vi "Init.vi"(8 "error in (no error)":errorcluster, 11 "uService Template in":refnum<class "DAQ Sender.lvclass">) -> (0 "error out":errorcluster, 3 "uService Template out":refnum<class "DAQ Sender.lvclass">)   [LabVIEW 2020, in "TALOS.lvlib" / "DAQ Sender.lvlib" / "DAQ Sender.lvclass"]
uses:
  DAQ Sender.lvclass
  C:/LabVIEW Code/TALOS/talos/Ancestor/Ancestor/Ancestor.lvclass
  C:/LabVIEW Code/TALOS/talos/Father of all uServices/Father of all uServices/Father of all uServices.lvclass
  Interfaces/DAQ Communication/DAQ Communication.lvclass
  Ancestor/Ancestor/Ancestor.lvclass/Ancestor.ctl
  Father of all uServices/Father of all uServices/Father of all uServices.lvclass/Father of all uServices.ctl
  DAQ Sender.lvclass/DAQ Sender.ctl
  Support VIs/Generate Error.vi
  FGV/Error Memory/Get Error Description.vi
  Support VIs/Get PC name.vi
  Support VIs/Get Class Name.vi
  <vilib>/Utility/error.llb/Clear Errors.vi
  FGV/Error Memory/Error Memory Core.vi
  <vilib>/AdvancedString/Delimited String to 1D String Array.vi
  Support VIs/Circus Root Path.vi
  FGV/Error Memory/Error Crt Lvl checker.vi
  FGV/Error Memory/Error Memory Core.vi/40c8088d-b597-4017-91af-faa98e00292e.vi
  FGV/Error Memory/Error Memory Core.vi/d4a3ab98-063c-4e44-b43d-fbdcfe6c2be2.vi
  Support VIs/Global Memory.vi
  <vilib>/Utility/LVClass/Get LV Class Name.vi
  Support VIs/Is in Packed Library.vi
  Support VIs/TALOS Root path.vi
  Support VIs/Read CSV worksheet.vi
  Support VIs/Global Constants.vi
  <vilib>/Utility/error.llb/General Error Handler.vi
  Support VIs/Error Log.vi
  <vilib>/Utility/config.llb/Open Config Data.vi
  <vilib>/Utility/config.llb/Get Section Names.vi
  <vilib>/Utility/config.llb/Get Key Names.vi
  <vilib>/Utility/config.llb/Read Key.vi
  <vilib>/Utility/config.llb/Read Key (String).vi
  <vilib>/Utility/config.llb/Close Config Data.vi
  <vilib>/Utility/error.llb/Search and Replace Pattern.vi
  Father of all uServices/Father of all uServices/Father of all uServices.lvclass
  Ancestor/Ancestor/Ancestor.lvclass
  <vilib>/Comparison/Equal/Equal Functor/Equal Functor.lvclass
  TALOS.lvlib
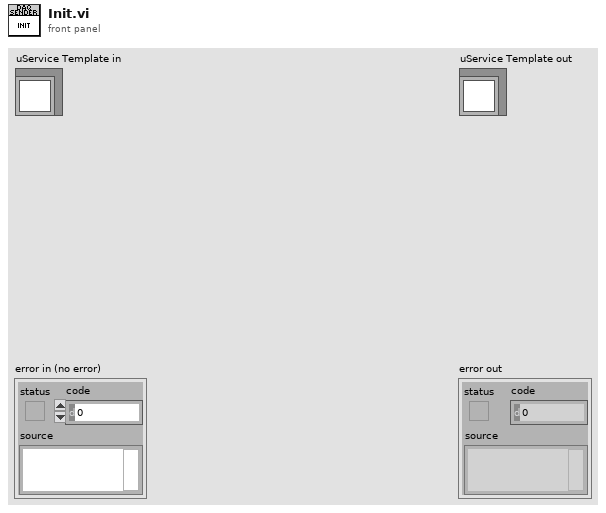
[diagram p1: front panel]
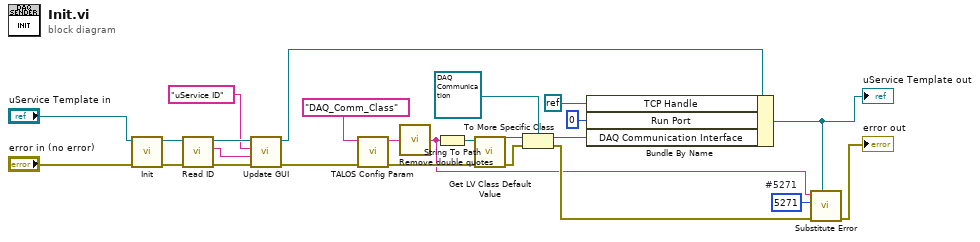
[diagram p0: block diagram]
diagram:
  w12 = 5271  # #5271
  n1 = call-parent "Init.vi"("error in (no error)"="error in (no error)", "uService Template in"="uService Template in") -> ("error out"=w21:errorcluster, "uService Template out"=w22:refnum<class "DAQ Sender.lvclass">)  [unwired: 8 in]
  n2 = call "Read ID.vi"("error in (no error)"=w21, "Ancestor in"=w22) -> ("error out"=w20:errorcluster, "ID"=w17:string, "Ancestor out"=w19:refnum<class "DAQ Sender.lvclass">)  [unwired: 7 in]
  n3 = call "Update GUI.vi"("error in (no error)"=w20, "Data"=w17, "GUI Item Name"="uService ID", "uService Template in"=w19) -> ("error out"=w1:errorcluster, "uService Template out"=w9:refnum<class "DAQ Sender.lvclass">)  [unwired: 6 in]
  n4 = call "TALOS Config Param.vi"("error in (no error)"=w1, "Parameter Name"="DAQ_Comm_Class") -> ("error out"=w25:errorcluster, "Output"=w2:string)  [unwired: 8 in]
  n5 = call "Remove double quotes.vi"("Input string"=w2) -> ("Output string"=w10:string)  [unwired: 4 in]
  n6 = String To Path(string=w10) -> (path=w16:path)
  n7 = call <vilib>:"Get LV Class Default Value.vi"("error in (no error)"=w25, "class path"=w16) -> ("error out"=w15:errorcluster, "object"=w14:refnum<class>)  [unwired: 8 in]
  n8 = To More Specific Class(target class=refnum<class "DAQ Communication.lvclass"> refnum ("DAQ Communication"), reference=w14, error in=w15) -> (specific class reference=w11:refnum<class "DAQ Communication.lvclass">, error out=w13:errorcluster)
  n9 = Bundle By Name(cluster=w9, "TCP Handle"=refnum<k0> refnum, "Run Port"=u16 0, "DAQ Communication Interface"=w11) -> (w7:refnum<class "DAQ Sender.lvclass">)
  "uService Template out" <- w7
  n10 = call "Substitute Error.vi"("LabVIEW Object"=w7, "error in (no error)"=w13, "Error Code"=w12, "Optional String"=w10) -> ("error out"=→"error out":errorcluster)  [unwired: 7 in]
